vi "LVDimInterface.test simple server.vi"() -> ()   [LabVIEW 2014, in "LVDimInterface.lvlib"]
doc: "This VI implements a DIM server, that publishes a loop counter as a DIM service"
uses:
  LVDimInterface.lvlib
panel:
  out "error out":errorcluster
  out "throughput [kBytes/s]":dbl
  out "updateRate [Hz]":dbl
  in  "nOfBuffers":i32=100
  in  "bufferSize":i32=10
  out "bufferCounter":i32
  in  "serverName":string="simpleServer"
  in  "serviceName":string="testBuffer"
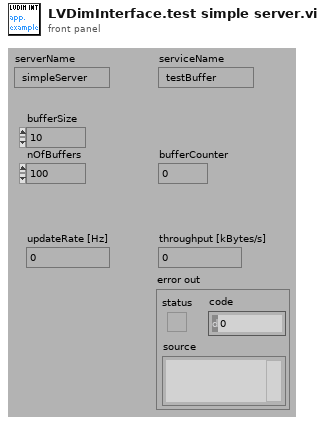
[diagram p1: front panel]
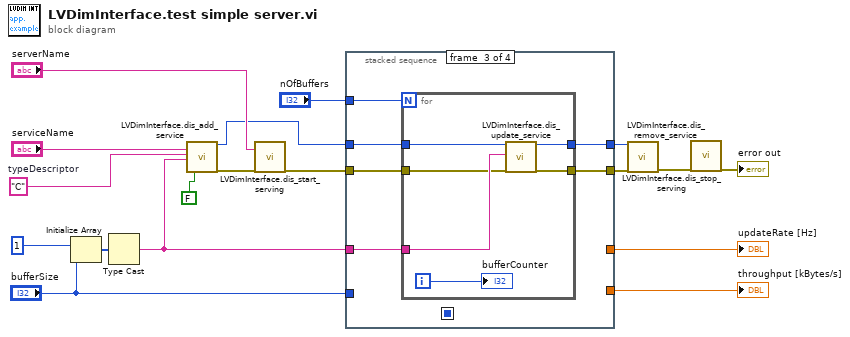
[diagram p0: block diagram]
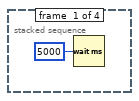
[diagram p2: hidden frame]
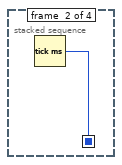
[diagram p3: hidden frame]
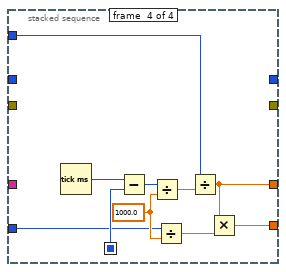
[diagram p4: hidden frame]
diagram:
  w11 = "C"  # typeDescriptor
  n1 = Initialize Array(i8 1 ("defaultData"), "bufferSize") -> (w8:i8[])
  n2 = Type Cast(x=w8) -> (*(type *) &x=w3:string)  [unwired: 1 in]
  n3 = call "LVDimInterface.dis_add_service.vi"("serviceName"="serviceName", "typeDescriptor"=w11, "data"=w3, "safeMode"=FALSE) -> ("my_serviceID"=w10:i32, "error out"=w17:errorcluster)  [unwired: 14 in]
  n4 = call "LVDimInterface.dis_start_serving.vi"("serverName"="serverName", "error in (no error)"=w17) -> ("error out"=w15:errorcluster)  [unwired: 16 in, 1 out]
  n5 = stacked-sequence {
    seq-local: [_ w20 _ _] -> [_ _ _ w41]
    tunnel: [_ _ w26 _] -> w18
    tunnel: w15 -> [_ _ w25 _]
    tunnel: [_ _ w24 _] -> w14
    tunnel: w10 -> [_ _ w23 _]
    tunnel: w3 -> [_ _ w22 _]
    tunnel: "nOfBuffers" -> [_ _ w21 w39]
    tunnel: "bufferSize" -> [_ _ _ w36]
    tunnel: [_ _ _ w34] -> w5
    tunnel: [_ _ _ w33] -> w4
    frame #0 {
      n6 = Wait (ms)(milliseconds to wait=u32 5000) -> ()  [unwired: 1 out]
    }
    frame #1 {
      n7 = Tick Count (ms)() -> (millisecond timer value=w20:u32)
    }
    frame #2 {
      n8 = for {
        N: w21 -> [_]
        tunnel: [w32] -> w26
        tunnel: w25 -> [w27]
        tunnel: [w30] -> w24
        tunnel: w23 -> [w28]
        tunnel: w22 -> [w29]
        i -> [w31]
        n9 = call "LVDimInterface.dis_update_service.vi"("my_serviceID"=w28, "data"=w29, "error in (no error)"=w27) -> ("my_serviceID out"=w32:i32, "error out"=w30:errorcluster)  [unwired: 14 in, 1 out]
        "bufferCounter" <- w31
      }
    }
    frame #3 {
      w37 = 1000.0 ("y")
      n10 = Tick Count (ms)() -> (millisecond timer value=w42:u32)
      n11 = Subtract(x=w42, y=w41) -> (x-y=w40:u32)
      n12 = Divide(x=w40, y=w37) -> (x/y=w38:dbl)
      n13 = Divide(x=w36, y=w37) -> (x/y=w35:dbl)
      n14 = Divide(x=w39, y=w38) -> (x/y=w34:dbl)
      n15 = Multiply(x=w34, y=w35) -> (x*y=w33:dbl)
    }
  }
  "updateRate [Hz]" <- w5
  "throughput [kBytes/s]" <- w4
  n16 = call "LVDimInterface.dis_remove_service.vi"("my_serviceID"=w18, "error in (no error)"=w14) -> ("error out"=w13:errorcluster)  [unwired: 17 in]
  n17 = call "LVDimInterface.dis_stop_serving.vi"("error in (no error)"=w13) -> ("error out"=→"error out":errorcluster)  [unwired: 18 in]
